vi "File_ToEasyObj.vi"(8 "error in (no error)":errorcluster, 11 "File in":refnum<class "File.lvclass">) -> (0 "error out":errorcluster, 2 "output cluster":T1 {"Groups"."Channels"."Data Reference" format="%.0x"}, 3 "File out":refnum<class "File.lvclass">)   [LabVIEW 2023, in "File.lvclass"]
doc: "Exports the current file definition to a data cluster. To be used when transferring the definition of our configured custom device between the System Explorer and Engine in VeriStand."
uses:
  File.lvclass
  FileAsCluster.ctl
  Group/GroupAsCluster.ctl
  Channel/ChannelAsCluster.ctl
  <vilib>/NI VeriStand/Custom Device API/Data Reference.ctl
  Meta Data.ctl
  File.lvclass/File.ctl
  Group/Group.lvclass
  <vilib>/NI VeriStand/Custom Device API/Custom Device API.lvlib
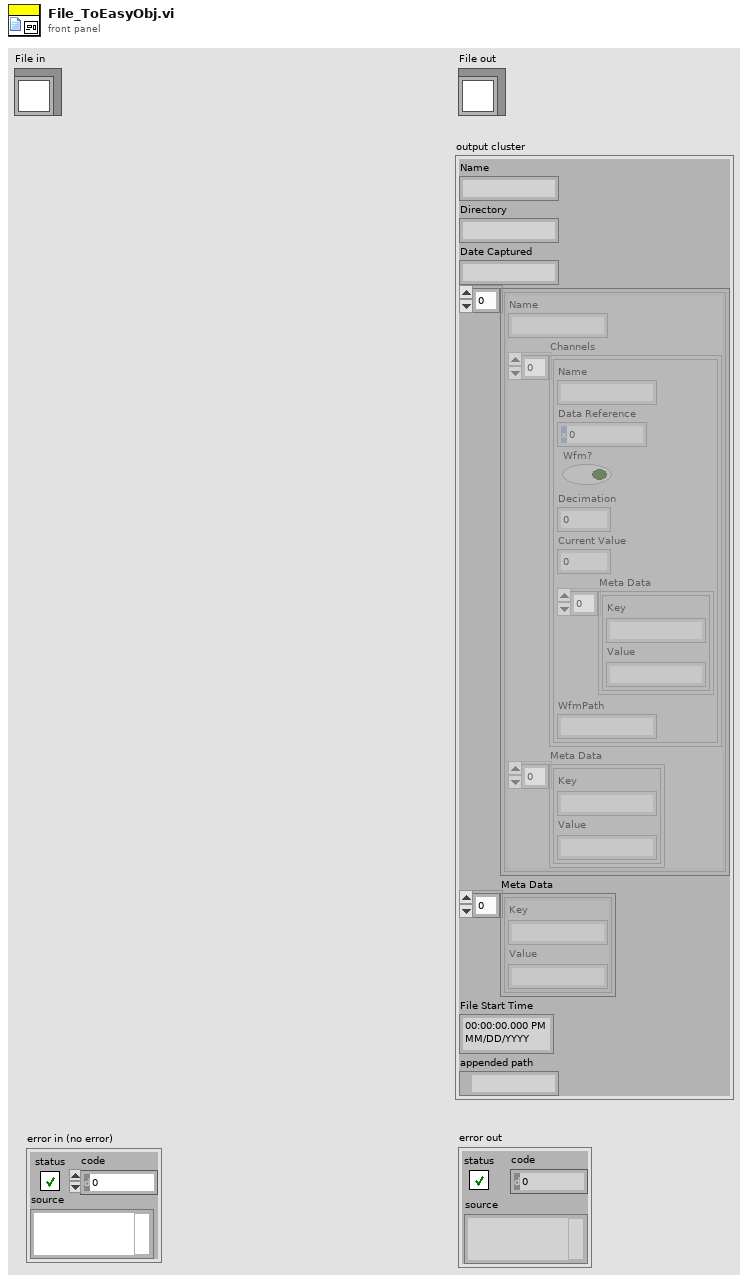
[diagram p1: front panel]
types:
  T1 = typedef "FileAsCluster.ctl" = cluster{"Name":string, "Directory":string, "Date Captured":string, "Groups":T2[], "Meta Data":T5[], "File Start Time":timestamp, "appended path":path}
  T2 = typedef "GroupAsCluster.ctl" = cluster{"Name":string, "Channels":T3[], "Meta Data":T5[]}
  T3 = typedef "ChannelAsCluster.ctl" = cluster{"Name":string, "Data Reference":T4, "Wfm?":bool, "Decimation":i32, "Current Value":dbl, "Meta Data":T5[], "WfmPath":string}
  T4 = typedef "Custom Device API.lvlib/Data Reference.ctl" = i32
  T5 = typedef "Meta Data.ctl" = cluster{"Key":string, "Value":string}
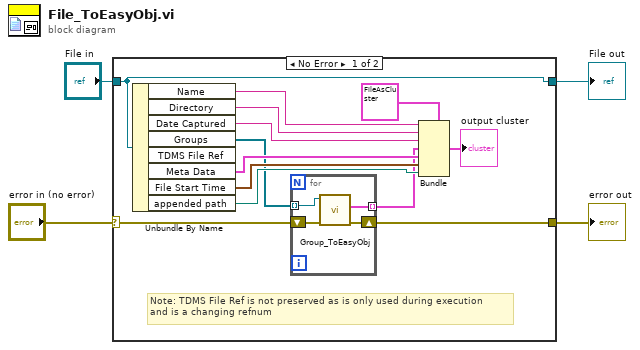
[diagram p0: block diagram]
diagram:
  n1 = case shown="No Error" "error in (no error)" {
    selector: "error in (no error)" -> [w9 w23]
    tunnel: [w8 w23] -> w3
    tunnel: [w17 w22] -> w1
    tunnel: "File in" -> [w17 w22]
    frame No Error {
      # "Note: TDMS File Ref is not preserved as is only used during execution\nand is a changing refnum"
      n2 = Unbundle By Name(w17) -> ("Name"=w16:string, "Directory"=w15:string, "Date Captured"=w14:string, "Groups"=w10:refnum<class "Group.lvclass">[], "Meta Data"=w13:T5[], "File Start Time"=w12:timestamp, "appended path"=w11:path)  [unwired: 1 out]
      n3 = for {
        tunnel: w10 -> [w21] mode=indexing
        shift-right: [w19] -> w8
        shift-left: w9 -> [w18]
        tunnel: [w20] -> w7 mode=indexing
        n4 = call-dynamic "Group_ToEasyObj.vi"("error in (no error)"=w18, "Group in"=w21) -> ("error out"=w19:errorcluster, "output cluster"=w20:T2)  [unwired: 7 in, 1 out]
      }
      n5 = Bundle(cluster=T1 {"Name"="", "Directory"="", "Date Captured"="", "Groups"=[], "Meta Data"=[], "File Start Time"=timestamp(0 s since 1904-01-01), "appended path"=path ""} ("output cluster"), "Name"=w16, "Directory"=w15, "Date Captured"=w14, "Groups"=w7, "Meta Data"=w13, "File Start Time"=w12, "appended path"=w11) -> (→"output cluster":T1)
    }
    frame Error {
    }
  }
  "error out" <- w3
  "File out" <- w1
